vi "BRig_generic_pathMove_pathInput.vi"(8 "input_error":errorcluster, 9 "input_Ioverwrite":bool, 10 "input_filePath_target":path, 11 "input_filePath_source":path) -> (0 "output_error":errorcluster, 1 "output_Iexist":bool, 2 "output_filePath_target":path)   [LabVIEW 2014]
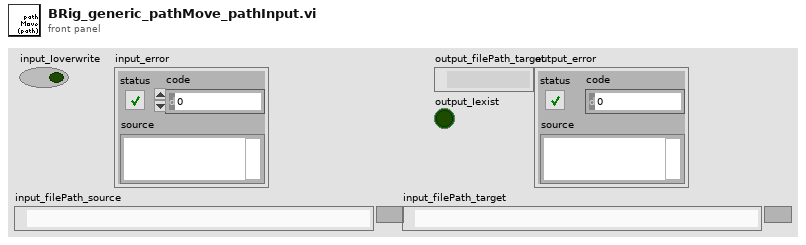
[diagram p1: front panel]
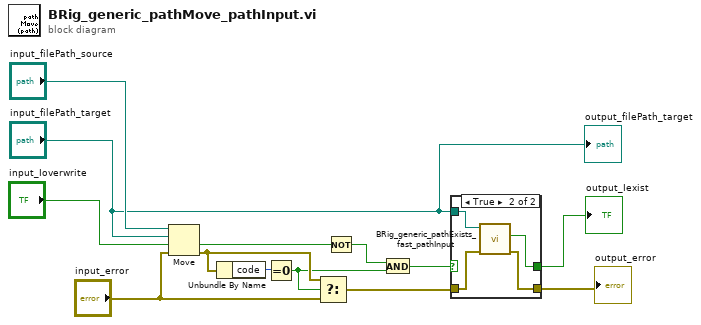
[diagram p0: block diagram]
diagram:
  n1 = Move(source path="input_filePath_source", error in="input_error", 9:"input_Ioverwrite", 10:"input_filePath_target") -> (error out=w11:errorcluster, 1:w8:bool)  [unwired: 1 in, 1 out]
  n2 = Unbundle By Name(w11) -> ("code"=w13:i32)
  n3 = Equal To 0?(x=w13) -> (x = 0?=w6:bool)
  n4 = Select(t=w11, s=w6, f="input_error") -> (s? t:f=w4:errorcluster)
  n5 = Not(x=w8) -> (.not. x?=w7:bool)
  n6 = And(x=w7, y=w6) -> (x .and. y?=w5:bool)
  n7 = case shown="True" w5 {
    selector: w5 -> [w14 _]
    tunnel: w4 -> [w15 w19]
    tunnel: "input_filePath_target" -> [_ w18]
    tunnel: [w15 w17] -> w2
    tunnel: [w14 w16] -> w1
    frame False {
    }
    frame True {
      n8 = call "BRig_generic_pathExists_fast_pathInput.vi"("input_error"=w19, "input_filePath"=w18) -> ("output_error"=w17:errorcluster, "output_Iexist"=w16:bool)  [unwired: 7 in, 1 out]
    }
  }
  "output_error" <- w2
  "output_Iexist" <- w1
  "output_filePath_target" <- "input_filePath_target"
